vi "calculate log time range.vi"(7 "Log Contents (\"\")":string) -> (2 "Log Stop Time":timestamp, 3 "Log Start Time":timestamp)   [LabVIEW 2011]
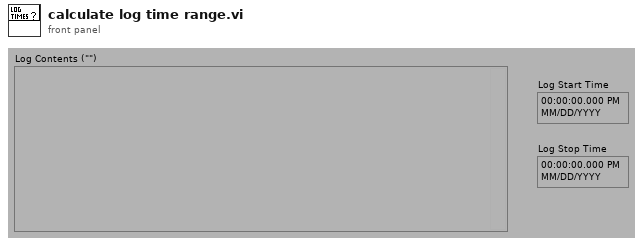
[diagram p1: front panel]
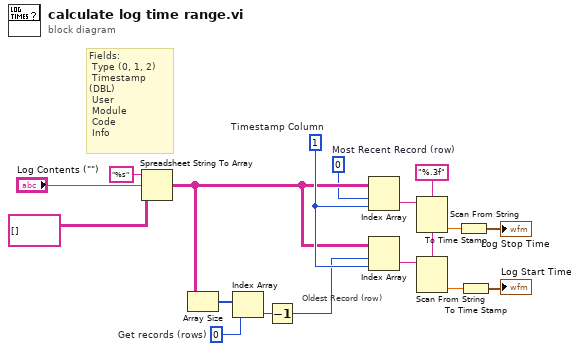
[diagram p0: block diagram]
diagram:
  w5 = 0  # Most Recent Record (row)
  w6 = 0  # Get records (rows)
  w12 = "%.3f"
  w16 = 1  # Timestamp Column
  # "Oldest Record (row)"
  # "Fields:\n Type (0, 1, 2)\n Timestamp (DBL)\n User\n Module\n Code\n Info"
  n1 = Spreadsheet String To Array(format string="%s", spreadsheet string="Log Contents (\"\")", array type (2D Dbl)=string[][] []) -> (array=w7:string[][])  [unwired: 1 out]
  n2 = Array Size(array=w7) -> (size(s)=w17:i32[])
  n3 = Index Array(array=w17, index=w6) -> (element=w15:i32)
  n4 = Decrement(x=w15) -> (x-1=w11:i32)
  n5 = Index Array(array=w7, index (row)=w5, index (col)=w16) -> (element=w14:string)
  n6 = Index Array(array=w7, index (row)=w11, index (col)=w16) -> (element=w13:string)
  n7 = Scan From String(format string=w12, input string=w14) -> (output 1=w4:dbl)  [unwired: 2 in, 4 out]
  n8 = Scan From String(format string=w12, input string=w13) -> (output 1=w3:dbl)  [unwired: 2 in, 4 out]
  n9 = To Time Stamp(1:w4) -> (0:→"Log Stop Time":timestamp)
  n10 = To Time Stamp(1:w3) -> (0:→"Log Start Time":timestamp)
